vi "K6514_InitializeCurrent.vi"(8 "error in (no error)":errorcluster, 10 "Range":dbl(ring)=0.02 items=["20 mA"=0.02, "2 mA"=0.002, "200 uA"=0.0002, "20 uA"=2e-05, "2 uA"=2e-06, "200 nA"=2e-07, "20 nA"=2e-08, "2 nA"=2e-09, "200 pA"=2e-10, "20 pA"=2e-11], 11 "VISA resource name":refnum<visa-resource-name>) -> (0 "error out":errorcluster, 3 "VISA resource name out":refnum<visa-resource-name>)   [LabVIEW 2024]
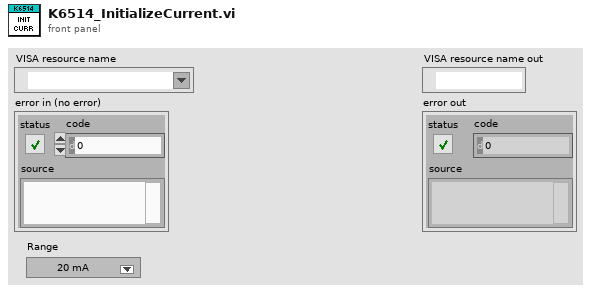
[diagram p1: front panel]
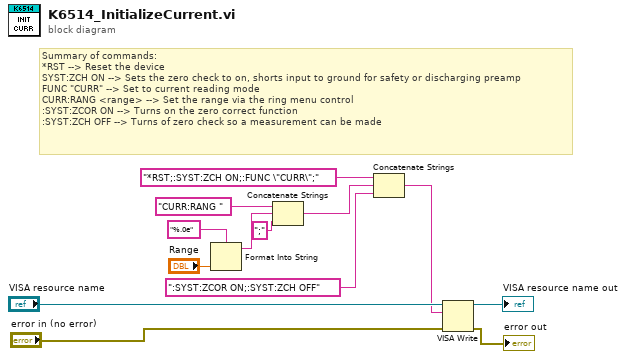
[diagram p0: block diagram]
diagram:
  # "Summary of commands:\n*RST --> Reset the device\nSYST:ZCH ON --> Sets the zero check to on, shorts input to ground for safety or discharging preamp\nFUNC \"CURR\" --> Set to current reading mode \nCURR:RANG <range> --> Set the range via the ring menu control \n:SYST:ZCOR ON --> Turns on the zero correct function\n:SYST:ZCH OFF --> Turns of zero check so a measurement can be made"
  n1 = Format Into String(format string="%.0e", "Range") -> (resulting string=w12:string)  [unwired: 2 in, 1 out]
  n2 = Concatenate Strings("CURR:RANG ", w12, ";" ("string")) -> (w3:string)
  n3 = Concatenate Strings("*RST;:SYST:ZCH ON;:FUNC \"CURR\";" ("write buffer"), w3, ":SYST:ZCOR ON;:SYST:ZCH OFF") -> (w1:string)
  n4 = VISA Write(VISA resource name="VISA resource name", write buffer=w1, error in (no error)="error in (no error)") -> (VISA resource name out=→"VISA resource name out":refnum<visa-resource-name>, error out=→"error out":errorcluster)  [unwired: 1 out]
